vi "visionMain.vi"(11 "camImage":T1) -> (0 "angle (deg)":dbl, 3 "distance (ft)":dbl)   [LabVIEW 2016]
uses:
  <vilib>/vision/Image Controls.llb/IMAQ Image.ctl
  Vision Support Code/Camera Types.ctl
  <vilib>/Rock Robotics/Network Tables/NT Read Number.vi
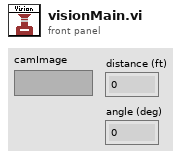
[diagram p1: front panel]
types:
  T1 = typedef "IMAQ Image.ctl" = refnum<image>
  T2 = cluster{"leftRight":dbl, "frontBack":dbl, "angle":dbl}
  T3 = cluster{"Hue":cluster{dbl, dbl}, "Sat":cluster{dbl, dbl}, "Val":cluster{dbl, dbl}}
  T4 = typedef "Camera Types.ctl" = enum16{"206", "1011", "1013", "MS HD3000 square", "MS HD3000 640x480"}
  T5 = cluster{cluster{"Numeric":dbl, "Numeric":dbl}, cluster{"Numeric":dbl, "Numeric":dbl}, cluster{"Numeric":dbl, "Numeric":dbl}}
  T6 = cluster{"Distance (ft)":dbl, "Score":dbl, "Normalized":cluster{"Center":cluster{dbl, dbl}, "Rectangle":cluster{"leftX":dbl, "topY":dbl, "rightX":dbl, "bottomY":dbl}}, "Pixels":cluster{"Center":cluster{dbl, dbl}, "Rectangle":cluster{"leftX":dbl, "topY":dbl, "rightX":dbl, "bottomY":dbl}}}
  T7 = cluster{"leftX":dbl, "topY":dbl, "rightX":dbl, "bottomY":dbl}
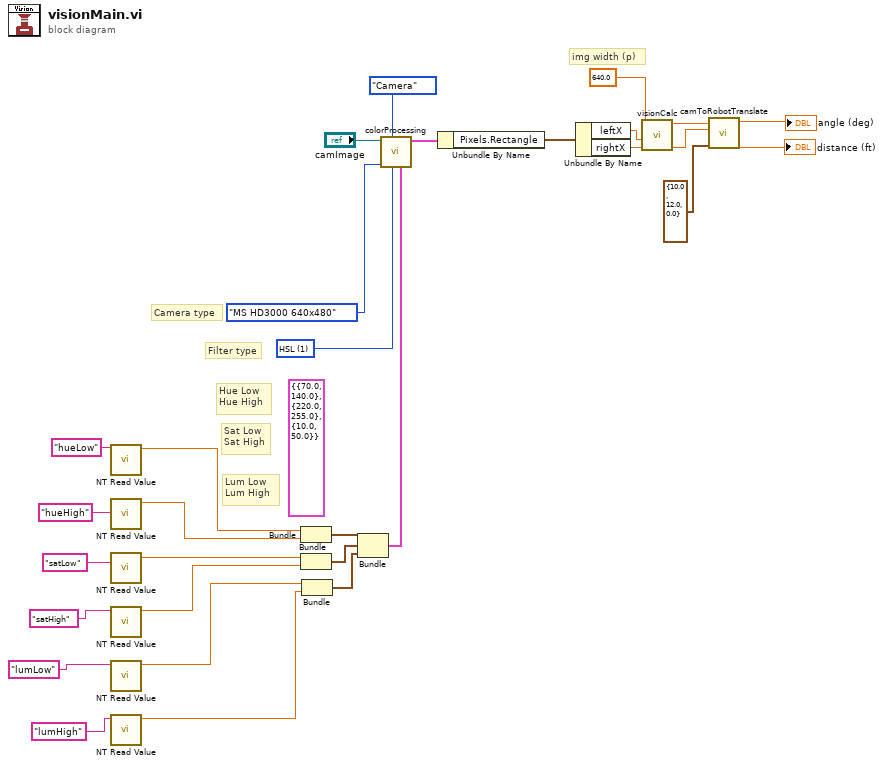
[diagram p0: block diagram]
diagram:
  (unwired) T3 {"Hue"={70.0, 140.0}, "Sat"={220.0, 255.0}, "Val"={10.0, 50.0}} ("LED Color")
  w25 = u16 1 items=["RGB", "HSL", "HSV", "HSI"] ("Color Mode")
  # "img width (p)"
  # "Lum Low\nLum High"
  # "Sat Low\nSat High"
  # "Hue Low\nHue High"
  # "Filter type"
  # "Camera type"
  n1 = call-poly <vilib>:"NT Read Value.vi"("Name"="hueLow") -> ("Numeric"=w19:dbl)  [unwired: 9 in, 1 out]
  n2 = call-poly <vilib>:"NT Read Value.vi"("Name"="hueHigh") -> ("Numeric"=w18:dbl)  [unwired: 9 in, 1 out]
  n3 = call-poly <vilib>:"NT Read Value.vi"("Name"="satLow") -> ("Numeric"=w17:dbl)  [unwired: 9 in, 1 out]
  n4 = call-poly <vilib>:"NT Read Value.vi"("Name"="satHigh") -> ("Numeric"=w16:dbl)  [unwired: 9 in, 1 out]
  n5 = call-poly <vilib>:"NT Read Value.vi"("Name"="lumLow") -> ("Numeric"=w15:dbl)  [unwired: 9 in, 1 out]
  n6 = call-poly <vilib>:"NT Read Value.vi"("Name"="lumHigh") -> ("Numeric"=w14:dbl)  [unwired: 9 in, 1 out]
  n7 = Bundle("Numeric"=w19, "Numeric"=w18) -> (w20:cluster{"Numeric":dbl, "Numeric":dbl})  [unwired: 1 in]
  n8 = Bundle("Numeric"=w17, "Numeric"=w16) -> (w21:cluster{"Numeric":dbl, "Numeric":dbl})  [unwired: 1 in]
  n9 = Bundle("Numeric"=w15, "Numeric"=w14) -> (w22:cluster{"Numeric":dbl, "Numeric":dbl})  [unwired: 1 in]
  n10 = Bundle(w20, w21, w22) -> (w13:T5)  [unwired: 1 in]
  n11 = call "colorProcessing.vi"("LED Color"=w13, "Color Mode"=w25, "Source"=enum32{"Files", "Camera"}."Camera", "Camera Type"=Camera_Types."MS HD3000 640x480", "camImage"="camImage") -> ("Results"=w26:T6)  [unwired: 6 in]
  n12 = Unbundle By Name(w26) -> ("Pixels.Rectangle"=w30:T7)
  n13 = Unbundle By Name(w30) -> ("leftX"=w29:dbl, "rightX"=w28:dbl)
  n14 = call "visionCalc.vi"("imgWidth"=640.0, "leftX"=w29, "rightX"=w28) -> ("angle (deg)"=w5:dbl, "distance (ft)"=w4:dbl)  [unwired: 6 in]
  n15 = call "camToRobotTranslate.vi"("camOffset"=T2 {"leftRight"=10.0, "frontBack"=12.0, "angle"=0.0}, "camDistToGoal"=w4, "camAngleToGoal"=w5) -> ("robotDistToGoal"=→"distance (ft)":dbl, "robotAngleToGoal"=→"angle (deg)":dbl)  [unwired: 7 in]
